vi "Resistance Parameters.vi"(0 "Data Management Control":T2, 2 "Specific Voltages 2":dbl[](array[numeric])=[32.0, 36.0], 5 "Selected Exp Settings":T3={"P2_Sweep_Stop_V"=36.0, "P2_Sweep_Step_V"=1.0, "Experiment Name"="", "Resistance Threshold"=1.0, "P1_Fixed_Voltage"=36.0, "P2_Sweep_Start_V"=36.0}, 7 "Voltage Calculated Values":T1, 11 "Error In":errorcluster) -> (4 "Resistance Calculated Values":T4, 6 "Resistance Array Calc":T5, 8 "TN4 Calc":T6, 15 "Error Out":errorcluster)   [LabVIEW 2013]
uses:
  Controls/Data Management.ctl
  Controls/Individual User Inputs.ctl
  Controls/Resistance Individual Calculated Values.ctl
  Controls/Resistance Array Calculated Values.ctl
  Controls/TN4 Calc.ctl
  Controls/Voltage Calculated Values.ctl
panel:
  in  "Tab Control":enum32{"Inputs", "Outputs"}(tab)
  out "Specific Voltages":dbl[](array[numeric])
  # "Test Settings"
  # "Make the Stop and Step Negative \nfor negative sweep"
  # "Calculation Settings"
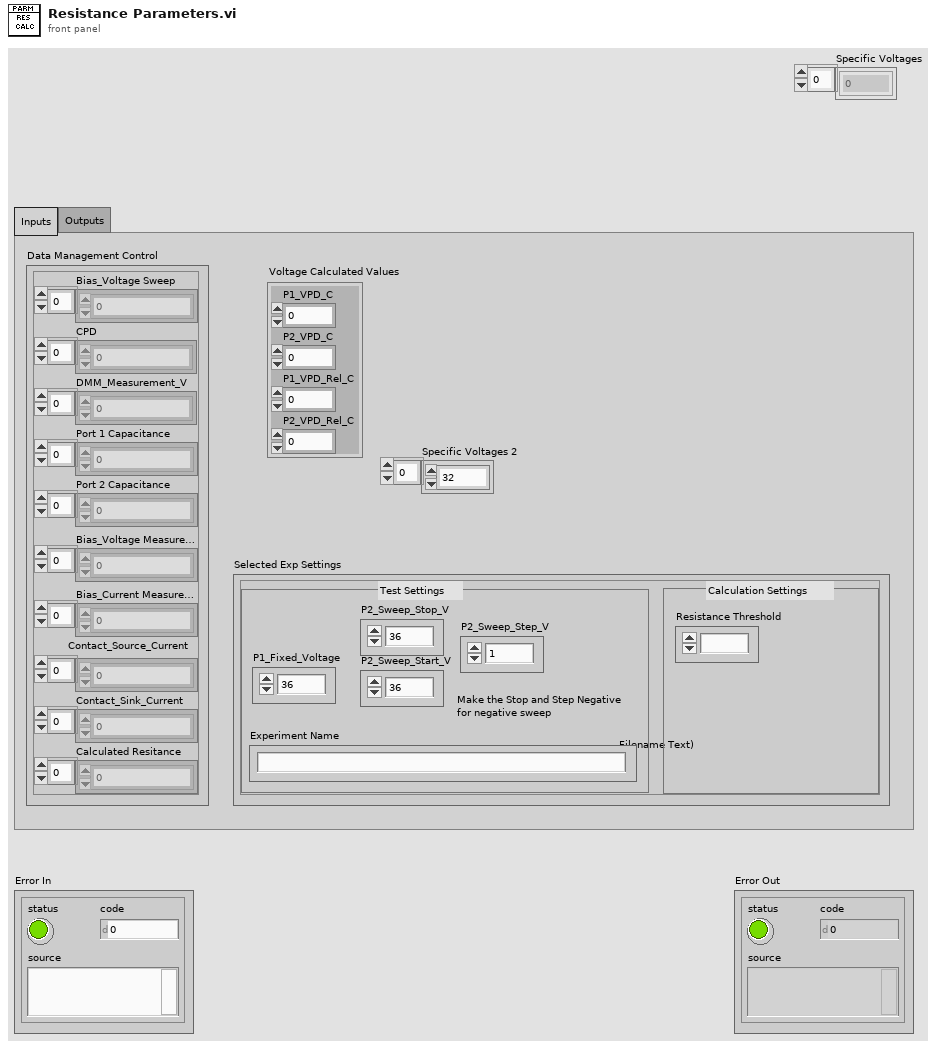
[diagram p1: front panel]
types:
  T1 = typedef "Voltage Calculated Values.ctl" = cluster{"P1_VPD_C":dbl, "P2_VPD_C":dbl, "P1_VPD_Rel_C":dbl, "P2_VPD_Rel_C":dbl}
  T2 = typedef "Data Management.ctl" = cluster{"Bias_Voltage Sweep":dbl[], "CPD":dbl[], "DMM_Measurement_V":dbl[], "Port 1 Capacitance":dbl[], "Port 2 Capacitance":dbl[], "Bias_Voltage Measurement":dbl[], "Bias_Current Measurement":dbl[], "Contact_Source_Current":dbl[], "Contact_Sink_Current":dbl[], "Calculated Resitance":dbl[]}
  T3 = typedef "Individual User Inputs.ctl" = cluster{"P2_Sweep_Stop_V":dbl, "P2_Sweep_Step_V":dbl, "Experiment Name":string, "Resistance Threshold":dbl, "P1_Fixed_Voltage":dbl, "P2_Sweep_Start_V":dbl}
  T4 = typedef "Resistance Individual Calculated Values.ctl" = cluster{"Rc_free":dbl, "Rc_first":dbl, "Rc_vmax":dbl, "Rc_last":dbl, "Rc_end":dbl, "VPD_R":dbl, "VPD_Rel_R":dbl}
  T5 = typedef "Resistance Array Calculated Values.ctl" = cluster{"RC@V":dbl[]}
  T6 = typedef "TN4 Calc.ctl" = cluster{"P1_TN4_ACT":dbl, "P2_TN4_ACT ":dbl, "VPD_R_2":dbl, "DVR":dbl}
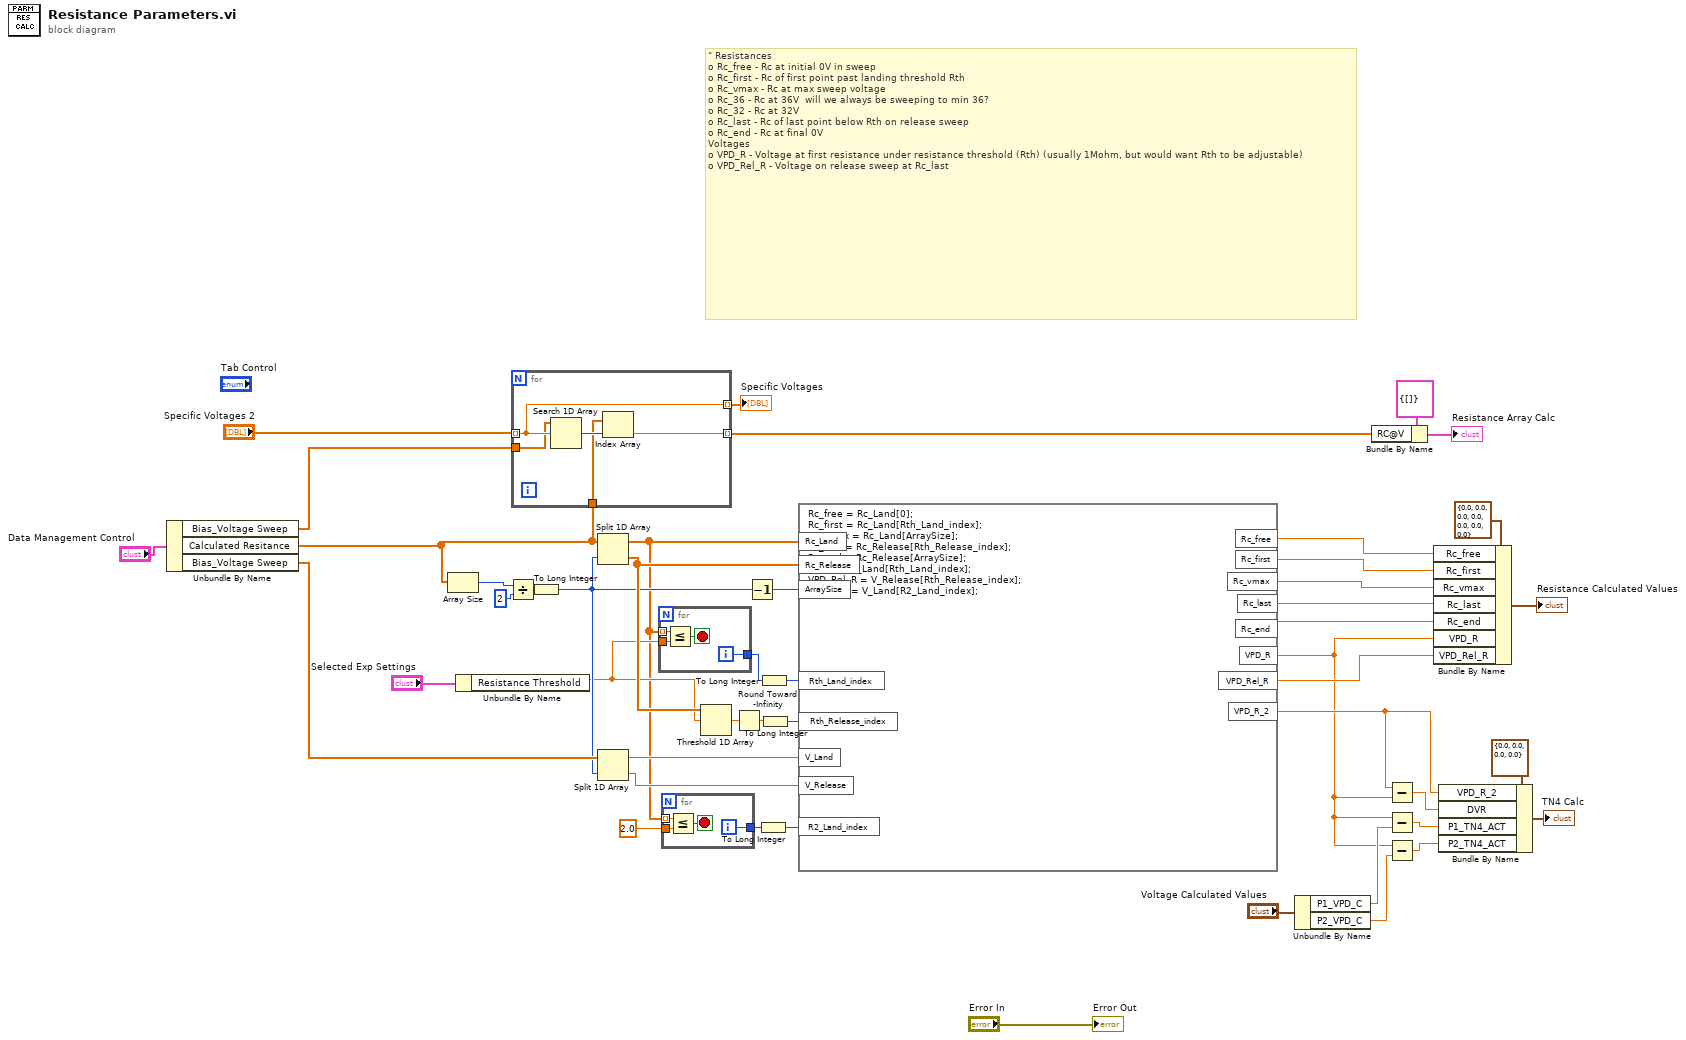
[diagram p0: block diagram]
diagram:
  # "\"\tResistances\no\tRc_free - Rc at initial 0V in sweep\no\tRc_first - Rc of first point past landing threshold Rth \no\tRc_vmax - Rc at max sweep voltage\no\tRc_36 - Rc at 36V  will we always be sweeping to min 36?\no\tRc_32 - Rc at 32V\no\tRc_last - Rc of last point below Rth on release sweep\no\tRc_end - Rc at final 0V\nVoltages\no\tVPD_R - Voltage at first resistance under resistance threshold (Rth) (usually 1Mohm, but would want Rth to be adjustable)\no\tVPD_Rel_R - Voltage on release sweep at Rc_last"
  n1 = Unbundle By Name("Data Management Control") -> ("Bias_Voltage Sweep"=w22:dbl[], "Calculated Resitance"=w16:dbl[], "Bias_Voltage Sweep"=w21:dbl[])
  n2 = Array Size(array=w16) -> (size(s)=w47:i32)
  n3 = Unbundle By Name("Selected Exp Settings") -> ("Resistance Threshold"=w18:dbl)
  n4 = Divide(x=w47, y=2) -> (x/y=w45:dbl)
  n5 = for {
    tunnel: "Specific Voltages 2" -> [w50] mode=indexing
    tunnel: [w51] -> w25 mode=indexing
    tunnel: [w50] -> w37 mode=indexing
    tunnel: w22 -> [w49]
    tunnel: w16 -> [w48]
    n6 = Search 1D Array(1D array=w49, element=w50) -> (index of element=w52:i32)  [unwired: 1 in]
    n7 = Index Array(array=w48, index=w52) -> (element=w51:dbl)
  }
  "Specific Voltages" <- w37
  n8 = To Long Integer(number=w45) -> (32bit integer=w20:i32)
  n9 = Split 1D Array(array=w16, index=w20) -> (first subarray=w12:dbl[], second subarray=w40:dbl[])
  n10 = Split 1D Array(array=w21, index=w20) -> (first subarray=w29:dbl[], second subarray=w28:dbl[])
  n11 = for {
    tunnel: [w56] -> w17
    tunnel: w12 -> [w55] mode=indexing
    tunnel: w18 -> [w54]
    i -> [w56]
    stop <- w53 stop-if-true
    n12 = Less Or Equal?(x=w55, y=w54) -> (x <= y?=w53:bool)
  }
  n13 = for {
    tunnel: [w60] -> w15
    tunnel: w12 -> [w59] mode=indexing
    tunnel: 2.0 ("Resistance Threshold") -> [w58]
    i -> [w60]
    stop <- w57 stop-if-true
    n14 = Less Or Equal?(x=w59, y=w58) -> (x <= y?=w57:bool)
  }
  n15 = Threshold 1D Array(2:w18, 3:w40) -> (0:w42:dbl)  [unwired: 1 in]
  n16 = Round Toward -Infinity(1:w42) -> (0:w41:dbl)
  n17 = Decrement(x=w20) -> (x-1=w19:i32)
  n18 = To Long Integer(number=w15) -> (32bit integer=w13:i32)
  n19 = To Long Integer(number=w17) -> (32bit integer=w43:i32)
  n20 = To Long Integer(number=w41) -> (32bit integer=w39:i32)
  n21 = formula code="Rc_free = Rc_Land[0];\nRc_first = Rc_Land[Rth_Land_index];\nRc_vmax = Rc_Land[ArraySize];\nRc_last = Rc_Release[Rth_Release_index];\nRc_end = Rc_Release[ArraySize];\nVPD_R = V_Land[Rth_Land_index];\nVPD_Rel_R = V_Release[Rth_Release_index];\nVPD_R_2 = V_Land[R2_Land_index];"("Rc_Land"=w12, "Rc_Release"=w40, "Rth_Land_index"=w43, "Rth_Release_index"=w39, "ArraySize"=w19, "V_Land"=w29, "V_Release"=w28, "R2_Land_index"=w13) -> ("Rc_free"=w35:dbl, "Rc_first"=w34:dbl, "Rc_vmax"=w33:dbl, "Rc_last"=w32:dbl, "Rc_end"=w31:dbl, "VPD_R"=w1:dbl, "VPD_Rel_R"=w9:dbl, "VPD_R_2"=w4:dbl)
  n22 = Unbundle By Name("Voltage Calculated Values") -> ("P1_VPD_C"=w6:dbl, "P2_VPD_C"=w3:dbl)
  n23 = Bundle By Name(cluster=T5 {"RC@V"=[]} ("Resistance Array Calc"), "RC@V"=w25) -> (→"Resistance Array Calc":T5)
  n24 = Subtract(x=w4, y=w1) -> (x-y=w8:dbl)
  n25 = Subtract(x=w1, y=w6) -> (x-y=w5:dbl)
  n26 = Subtract(x=w1, y=w3) -> (x-y=w2:dbl)
  n27 = Bundle By Name(cluster=T4 {"Rc_free"=0.0, "Rc_first"=0.0, "Rc_vmax"=0.0, "Rc_last"=0.0, "Rc_end"=0.0, "VPD_R"=0.0, "VPD_Rel_R"=0.0} ("Resistance Calculated Values"), "Rc_free"=w35, "Rc_first"=w34, "Rc_vmax"=w33, "Rc_last"=w32, "Rc_end"=w31, "VPD_R"=w1, "VPD_Rel_R"=w9) -> (→"Resistance Calculated Values":T4)
  n28 = Bundle By Name(cluster=T6 {"P1_TN4_ACT"=0.0, "P2_TN4_ACT "=0.0, "VPD_R_2"=0.0, "DVR"=0.0} ("TN4 Calc"), "VPD_R_2"=w4, "DVR"=w8, "P1_TN4_ACT"=w5, "P2_TN4_ACT"=w2) -> (→"TN4 Calc":T6)
  "Error Out" <- "Error In"
